vi "Commit.vi"(7 "Data":variant, 8 "error in (no error)":errorcluster, 9 "UUID":string, 10 "Dataset":string, 11 "CubeLogger in":refnum<class "CubeLogger.lvclass">) -> (0 "error out":errorcluster, 3 "CubeLogger out":refnum<class "CubeLogger.lvclass">, 4 "Replaced?":bool, 6 "Ready?":bool)   [LabVIEW 2018, in "CubeLogger.lvclass"]
uses:
  CubeLogger.lvclass
  CubeLogger.lvclass/CubeLogger.ctl
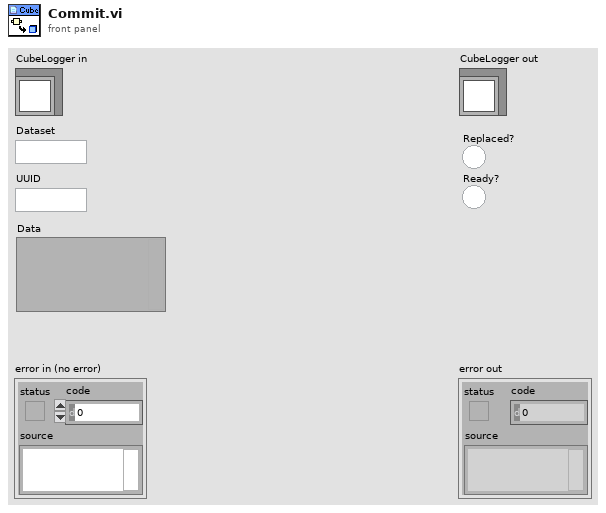
[diagram p1: front panel]
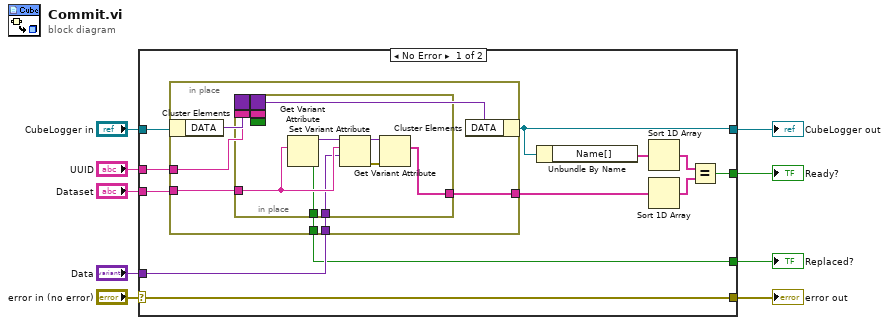
[diagram p0: block diagram]
diagram:
  n1 = case shown="No Error" "error in (no error)" {
    selector: "error in (no error)" -> [w21 w39]
    tunnel: [w21 w39] -> w8
    tunnel: [w15 w38] -> w6
    tunnel: "CubeLogger in" -> [w20 w38]
    tunnel: "UUID" -> [w19 _]
    tunnel: "Dataset" -> [w18 _]
    tunnel: "Data" -> [w17 _]
    tunnel: [w16 _] -> w2
    tunnel: [w10 _] -> w1
    frame No Error {
      n2 = in-place {
        in-place-border: w19 -> [w27]
        in-place-border: w18 -> [w26]
        in-place-border: [w24] -> w16
        in-place-border: w17 -> [w23]
        in-place-border: [w22] -> w13
        n3 = in-place-cluster #1(w20) -> ("DATA"=w28:variant)
        n4 = in-place {
          in-place-border: w26 -> [w36]
          in-place-border: [w35] -> w24
          in-place-border: w23 -> [w34]
          in-place-border: [w29] -> w22
          border: w28 -> [_]
          border: w27 -> [_]
          border: [_] -> w25
          border: _ -> [_]
          border: _ -> [_]
          n5 = Get Variant Attribute(Variant=w37, name=w36) -> (duplicate Variant=w33:variant, found=w35:bool)  [unwired: 2 in, 2 out]
          n6 = Set Variant Attribute(Variant=w33, name=w36, value=w34) -> (Variant out=w31:variant, error out=w32:errorcluster)  [unwired: 1 in, 1 out]
          n7 = Get Variant Attribute(Variant=w31, error in=w32) -> (duplicate Variant=w30:variant, names=w29:string[])  [unwired: 2 in, 2 out]
        }
        n8 = in-place-cluster #1("DATA"=w25) -> (w15:refnum<class "CubeLogger.lvclass">)
      }
      n9 = Unbundle By Name(w15) -> ("Name[]"=w14:string[])
      n10 = Sort 1D Array(array=w14) -> (sorted array=w12:string[])
      n11 = Sort 1D Array(array=w13) -> (sorted array=w11:string[])
      n12 = Equal?(x=w12, y=w11) -> (x = y?=w10:bool)
    }
    frame Error {
    }
  }
  "error out" <- w8
  "CubeLogger out" <- w6
  "Replaced?" <- w2
  "Ready?" <- w1
